vi "OAT Easy Gabor Spectral Map (Digital Tach).vi"(0 "scaled signal [EU]":waveform(dbl)={"t0"=timestamp(0 s since 1904-01-01), "dt"=0.0, "Y"=[]}, 1 "dB On (T)":bool=TRUE, 7 "digital tach info":T6={"tacho counts"=[], "counter timebase [Hz]"=20000000.0, "counter task type"=enum."event counting", "counter digit (32)"=32}, 9 "pulse/revolution (1)":i32=1, 11 "error in (no error)":errorcluster, 12 "type":T5(ring)=enum."RPM-Order", 13 "window info in (auto)":T1={"window type"=10, "window length"=0} {"window type" items=["None"=0, "Hanning"=1, "Hamming"=2, "Blackman-Harris"=3, "Exact Blackman"=4, "Blackman"=5, "Flat Top"=6, "4 Term B-Harris"=7, "7 Term B-Harris"=8, "Low Sidelobe"=9, "Gaussian"=62]; "window length" min=0}) -> (3 "speed profile":T2 {"speed [RPM]" format="%.2f"; "time [s]" format="%.2f"}, 4 "spectral map":dbl[][](array[numeric]) format="%.2f", 6 "scales":T4 {"Y scale"."multiplier" format="%.2f"; "Y scale"."offset" format="%.2f"; "X scale"."multiplier" format="%.2f"; "X scale"."offset" format="%.2f"}, 8 "unit labels":T3, 15 "error out":errorcluster)   [LabVIEW 2017]
doc: "Returns the spectral map of <B>scaled signal [EU]</B>. You can use this polymorphic VI to obtain a spectral map for an analog tachometer signal or a digital tachometer signal. The data type you wire to the <B>analog tach signal</B> input determines the polymorphic instance to use."
uses:
  <vilib>/addons/Sound and Vibration/Order Analysis/Tach Process/SubVIs/digital tach info.ctl
  <vilib>/addons/Sound and Vibration/Order Analysis/Tach Process/SubVIs/speed profile.ctl
  <vilib>/addons/Sound and Vibration/Order Analysis/Ref Gabor Order Tracking/window information.ctl
  <vilib>/addons/Sound and Vibration/Order Analysis/Backward Compatibility/Get Spectral Map (DBL).vi
  <vilib>/addons/Sound and Vibration/Order Analysis/Tach Process/SoundVib_TachProcess.lvlib
  <vilib>/addons/Sound and Vibration/Order Analysis/Gabor Order Tracking/SoundVib_Gabor.lvlib
panel:
  # "OAT Easy Gabor Spectral Map (Digital Tach)"
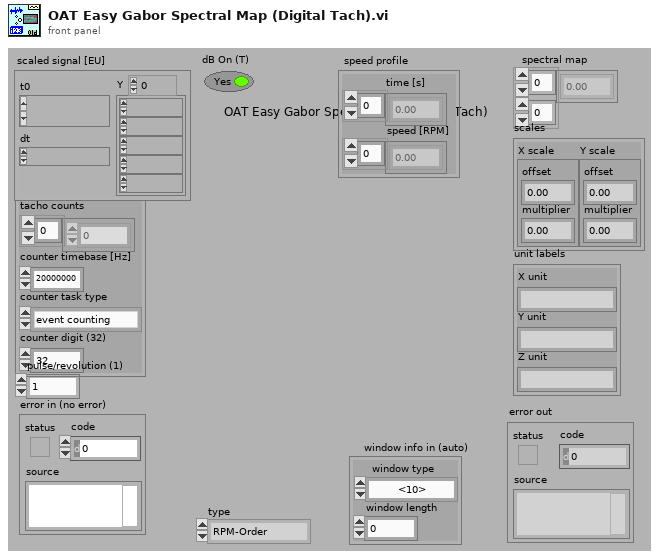
[diagram p1: front panel]
types:
  T1 = typedef "SoundVib_Gabor.lvlib/window information.ctl" = cluster{"window type":u32, "window length":i32}
  T2 = typedef "SoundVib_TachProcess.lvlib/speed profile.ctl" = cluster{"time [s]":dbl[], "speed [RPM]":dbl[]}
  T3 = cluster{"X unit":string, "Y unit":string, "Z unit":string}
  T4 = cluster{"X scale":cluster{"offset":dbl, "multiplier":dbl}, "Y scale":cluster{"offset":dbl, "multiplier":dbl}}
  T5 = enum16{"Frequency-Time", "Frequency-RPM", "Order-RPM", "RPM-Order"}
  T6 = typedef "SoundVib_TachProcess.lvlib/digital tach info.ctl" = cluster{"tacho counts":i64[], "counter timebase [Hz]":dbl, "counter task type":enum16{"period measurement", "event counting"}, "counter digit (32)":i32}
  T7 = cluster{"X scale":cluster{"offset":dbl, "multiplier":dbl}, "Y scale":cluster{"offset":dbl, "multiplier":dbl}, "Z scale":cluster{"offset":dbl, "multiplier":dbl}}
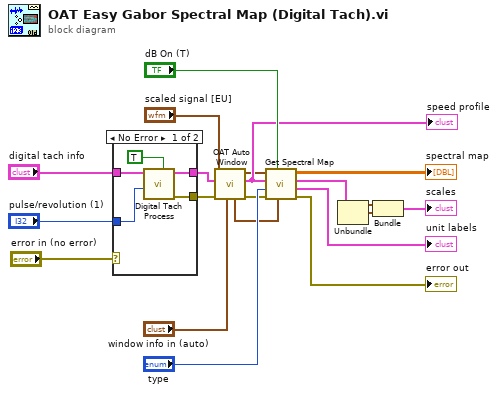
[diagram p0: block diagram]
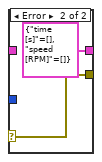
[diagram p2: hidden frame]
diagram:
  n1 = case shown="No Error" "error in (no error)" {
    selector: "error in (no error)" -> [_ w26]
    tunnel: "digital tach info" -> [w25 _]
    tunnel: "pulse/revolution (1)" -> [w24 _]
    tunnel: [w23 T2 {"time [s]"=[], "speed [RPM]"=[]} ("speed profile")] -> w6
    tunnel: [w22 w26] -> w3
    frame No Error {
      n2 = call <vilib>:"Digital Tach Process.vi"("reset? (True)"=TRUE ("reset? (False)"), "pulse/revolution (1)"=w24, "digital tach info"=w25) -> ("error out"=w22:errorcluster, "speed profile"=w23:T2)  [unwired: 6 in, 1 out]
    }
    frame Error {
    }
  }
  n3 = call <vilib>:"OAT Auto Window.vi"("window info in"="window info in (auto)", "error in (no error)"=w3, "speed profile"=w6, "scaled signal [EU]"="scaled signal [EU]") -> ("error out"=w2:errorcluster, "speed profile out"=w14:T2, "scaled signal [EU] out"=w5:waveform(dbl), "window info out"=w4:T1)  [unwired: 4 in]
  "speed profile" <- w14
  n4 = call-poly <vilib>:"Get Spectral Map.vi"("window info"=w4, "dB On (T)"="dB On (T)", "error in (no error)"=w2, "type"="type", "speed profile"=w14, "scaled signal [EU]"=w5) -> ("error out"=→"error out":errorcluster, "unit labels"=→"unit labels":T3, "scales"=w9:T7, "spectral map"=→"spectral map":dbl[][])  [unwired: 1 in, 1 out]
  n5 = Unbundle(w9) -> ("X scale"=w8:cluster{"offset":dbl, "multiplier":dbl}, "Y scale"=w7:cluster{"offset":dbl, "multiplier":dbl})  [unwired: 1 out]
  n6 = Bundle("X scale"=w8, "Y scale"=w7) -> (→"scales":T4)  [unwired: 1 in]
